vi "dfd_NStage MRate Filter Design with CIC.vi"(4 "filtering mode":T8=2 items=["No Rate Change", "Interpolation", "Decimation"], 6 "fs [Hz]":dbl=1000.0, 8 "error in (no error)":errorcluster, 9 "ripple specs":T1={"passband"=0.03624968728875148, "stopband"=0.001, "dB/linear? (T: dB)"=FALSE}, 10 "freq spec":T2={"fpass"=55.0, "fstop"=70.0}, 11 "CIC factor":i32=2) -> (0 "error out":errorcluster, 3 "multirate filters out":T3[](array[typedef]) {"mMRate_SumWl" min=1 max=32 step=1; "mMRate_InputIwl" min=1 max=32 step=1; "mMRate_GainWl" min=1 max=32 step=1; "mMRate_OutputWl" min=1 max=32 step=1; "mMRate_InputWl" min=1 max=32 step=1; "mMRate_CoefWl" min=1 max=32 step=1; "mMRate_Mode" items=["Default"=-1, "No Rate Change"=0, "Interpolation"=1, "Decimation"=2, "Interpolated"=3, "Rational"=4]})   [LabVIEW 2017, in "NI_DigFilterLicensed.lvlib"]
uses:
  <vilib>/addons/Digital Filter Design/NI_DigFilterLicensed.lvlib
  <vilib>/addons/Digital Filter Design/_Objects.llb/DFD Multirate Filtering Mode.ctl
  <vilib>/addons/Digital Filter Design/_Objects.llb/DFD Multirate Filter Obj.ctl
  <vilib>/addons/Digital Filter Design/_Objects.llb/DFD Multirate Mode.ctl
  <vilib>/addons/Digital Filter Design/_Objects.llb/DFD Coef Norm Type.ctl
  <vilib>/addons/Digital Filter Design/_Objects.llb/DFD Round-off Mode.ctl
  <vilib>/addons/Digital Filter Design/_Objects.llb/DFD FXP MRate Multiply Mode.ctl
  <vilib>/addons/Digital Filter Design/_Objects.llb/DFD Multirate Filter Specification (Design).ctl
  <vilib>/addons/Digital Filter Design/_Objects.llb/DFD Filter Ripple Specification (Design).ctl
  <vilib>/addons/Digital Filter Design/NI_DigFilter_Process.lvlib
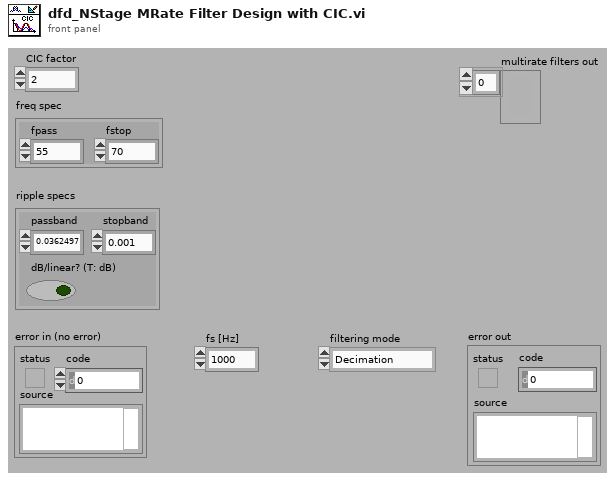
[diagram p1: front panel]
types:
  T1 = typedef "NI_DigFilterLicensed.lvlib/DFD Filter Ripple Specification (Design).ctl" = cluster{"passband":dbl, "stopband":dbl, "dB/linear? (T: dB)":bool}
  T2 = typedef "NI_DigFilterLicensed.lvlib/DFD Multirate Filter Specification (Design).ctl" = cluster{"fpass":dbl, "fstop":dbl}
  T3 = typedef "NI_DigFilterLicensed.lvlib/DFD Multirate Filter Obj.ctl" = cluster{"mMRate_Structure":enum16{"CIC", "FIR", "IIR", "Lattice"}, "mMRate_Mode":T4, "mMRate_Factor":i32, "mMRate_FIRParams":cluster{"mMRate_FIR_H":dbl[], "mMRate_FIR_IsNyquist?":bool, "mMRate_FIR_IsSymmetric?":bool}, "mMRate_CICParams":cluster{"mMRate_CIC_#Stage":i32, "mMRate_CIC_Lag":i32, "mMRate_CIC_Type":enum16{"Lowpass", "Highpass"}}, "mMRate_Order":i32, "mMRate_Version":string, "mMRate_Comments":string, "mMRate_RationalFactor":cluster{"mMRate_L":i32, "mMRate_M":i32}, "mMRate_Fs":dbl, "mMRate_Quantized?":bool, "mMRate_QFilterGain":dbl, "mMRate_CoefWl":i16, "mMRate_Scaling":cluster{"mMRate_ScaleByPowerOf2?":bool, "mMRate_ScaleType":T5}, "mMRate_InputWl":i16, "mMRate_OutputWl":i16, "mMRate_OutputMode":T6, "mMRate_MultMode":T7, "mMRate_BitPruning":bool, "mMRate_GainWl":i16, "mMRate_OutputFwl":i16, "mMRate_SumIwl":i16, "mMRate_InputIwl ":i16, "mMRate_SumWl":i16, "mMRate_CoefIwl":i16}
  T4 = typedef "NI_DigFilterLicensed.lvlib/DFD Multirate Mode.ctl" = i16
  T5 = typedef "NI_DigFilterLicensed.lvlib/DFD Coef Norm Type.ctl" = enum16{"No Norm", "Time Domain 1-Norm", "Time Domain 2-Norm", "Time Domain Inf-Norm"}
  T6 = typedef "NI_DigFilterLicensed.lvlib/DFD Round-off Mode.ctl" = enum16{"Nearest", "Truncation"}
  T7 = typedef "NI_DigFilterLicensed.lvlib/DFD FXP MRate Multiply Mode.ctl" = enum16{"Truncated", "Full"}
  T8 = typedef "NI_DigFilterLicensed.lvlib/DFD Multirate Filtering Mode.ctl" = u16
  T9 = typedef "NI_DigFilterLicensed.lvlib/DFD Filter Obj.ctl" = cluster{"mSRate_Fs":dbl, "mSRate_Version":string, "mSRate_Comments":string, "mSRate_OrgCoef":T10, "mSRate_CurCoef":T10, "mSRate_Quantized?":bool, "mSRate_QCoef":T10, "mSRate_QSettings":T12[], "mSRate_Order":i32, "mSRate_Scaling":cluster{"mSRate_ScaleByPowerOf2?":bool, "mSRate_ScaleType":T5}}
  T10 = typedef "NI_DigFilterLicensed.lvlib/DFD Filter Coef.ctl" = cluster{"type":T11, "gain":dbl, "coef a (k)":dbl[], "coef b (v)":dbl[]}
  T11 = typedef "NI_DigFilterLicensed.lvlib/DFD Filter Structure Type Selector.ctl" = enum16{"Undefined", "FIR Direct Form", "FIR Direct Form Transposed", "FIR Symmetric", "FIR Antisymmetric", "IIR Direct Form I", "IIR Direct Form I Transposed", "IIR Direct Form II", "IIR Direct Form II Transposed", "IIR Cascaded Second Order Sections Form I", "IIR Cascaded Second Order Sections Form I Transposed", "IIR Cascaded Second Order Sections Form II", "IIR Cascaded Second Order Sections Form II Transposed", "Lattice Allpass (basic sections)", "Lattice Allpass (one multiplier sections)", "Lattice Allpass (normalized sections)", "Lattice AR (basic sections)", "Lattice AR (one multiplier sections)", "Lattice AR (normalized sections)", "Lattice MA (minimum phase)", "Lattice MA (maximum phase)", "Lattice ARMA (basic sections)", "Lattice ARMA (one multiplier sections)", "Lattice ARMA (normalized sections)"}
  T12 = typedef "NI_DigFilterLicensed.lvlib/dfd_Internal Quantization Settings.ctl" = cluster{"source":T13, "wl":i16, "iwl":i16, "overflow mode":enum16{"Saturation", "Wrap"}, "rounding mode":enum16{"Nearest", "Truncation"}, "signed?":bool}
  T13 = typedef "NI_DigFilterLicensed.lvlib/dfd_Internal Quantization Srcs.ctl" = u16
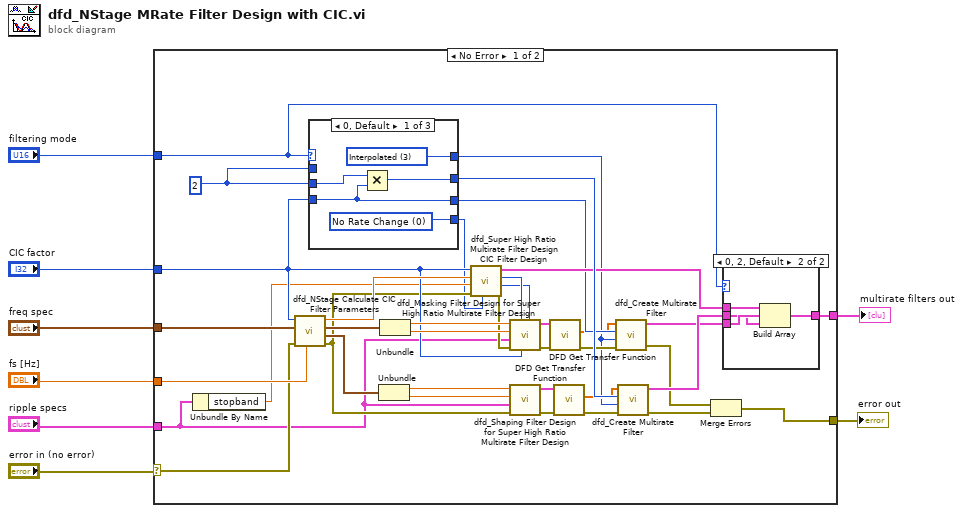
[diagram p0: block diagram]
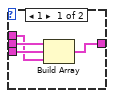
[diagram p2: hidden frame]
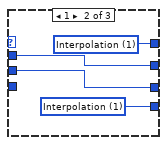
[diagram p3: hidden frame]
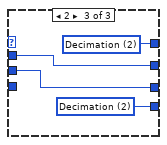
[diagram p4: hidden frame]
diagram:
  n1 = case shown="No Error" "error in (no error)" {
    selector: "error in (no error)" -> [w29 w68]
    tunnel: "fs [Hz]" -> [w46 _]
    tunnel: "ripple specs" -> [w10 _]
    tunnel: "filtering mode" -> [w32 _]
    tunnel: [w31 _] -> w7
    tunnel: "CIC factor" -> [w30 _]
    tunnel: [w17 w68] -> w4
    tunnel: "freq spec" -> [w14 _]
    frame No Error {
      w13 = 2 ("CIC factor")
      n2 = Unbundle By Name(w10) -> ("stopband"=w11:dbl)
      n3 = call <vilib>:"dfd_NStage Calculate CIC Filter Parameters.vi"("fs [Hz]"=w46, "error in (no error)"=w29, "freq spec"=w14, "CIC factor"=w30) -> ("error out"=w12:errorcluster, "shaping para"=w45:cluster{"fpass":dbl, "stop":dbl}, "masking para"=w38:cluster{"fpass":dbl, "fstop":dbl}, "CIC fstop"=w40:dbl)  [unwired: 2 in, 2 out]
      n4 = case shown="0, Default" w32 {
        tunnel: w13 -> [_ w62 w67]
        tunnel: [w57 w62 w67] -> w41
        tunnel: w13 -> [w58 w63 w66]
        tunnel: [w59 w63 w66] -> w26
        tunnel: [w55 w60 w64] -> w9
        tunnel: w30 -> [w59 _ _]
        tunnel: [w56 w61 w65] -> w21
        frame 0, Default {
          w55 = T8 0 items=["No Rate Change", "Interpolation", "Decimation"] ("filtering mode")
          w56 = T4 3 items=["Default"=-1, "No Rate Change"=0, "Interpolation"=1, "Decimation"=2, "Interpolated"=3] ("mode")
          n5 = Multiply(x=w58, y=w59) -> (x*y=w57:i32)
        }
        frame 1 {
          w60 = T8 1 items=["No Rate Change", "Interpolation", "Decimation"] ("filtering mode")
          w61 = T4 1 items=["Default"=-1, "No Rate Change"=0, "Interpolation"=1, "Decimation"=2, "Interpolated"=3] ("mode")
        }
        frame 2 {
          w64 = T8 2 items=["No Rate Change", "Interpolation", "Decimation"] ("filtering mode")
          w65 = T4 2 items=["Default"=-1, "No Rate Change"=0, "Interpolation"=1, "Decimation"=2, "Interpolated"=3] ("mode")
        }
      }
      n6 = Unbundle(w45) -> ("fpass"=w44:dbl, "stop"=w43:dbl)
      n7 = Unbundle(w38) -> ("fpass"=w37:dbl, "fstop"=w36:dbl)
      n8 = call <vilib>:"dfd_Super High Ratio Multirate Filter Design CIC Filter Design.vi"("filtering mode"=w9, "error in (no error)"=w12, "stop band attenuation [dB]"=w11, "fstop"=w40, "CIC factor"=w30) -> ("error out"=w28:errorcluster, "CIC order"=w15:i32, "CIC stage"=w39:i32, "multirate filter out"=w35:T3)  [unwired: 1 in, 2 out]
      n9 = call <vilib>:"dfd_Masking Filter Design for Super High Ratio Multirate Filter Design.vi"("CIC order"=w15, "CIC factor"=w30, "CIC stage"=w39, "error in (no error)"=w28, "ripple specs"=w10, "fstop"=w36, "fpass"=w37) -> ("error out"=w20:errorcluster, "filter out"=w24:T9)  [unwired: 1 in, 2 out]
      n10 = call <vilib>:"dfd_Shaping Filter Design for Super High Ratio Multirate Filter Design.vi"("error in (no error)"=w12, "ripple specs"=w10, "fstop"=w43, "fpass"=w44) -> ("error out"=w19:errorcluster, "filter out"=w42:T9)  [unwired: 1 in, 5 out]
      n11 = call <vilib>:"DFD Get Transfer Function.vi"("error in (no error)"=w20, "filter in"=w24) -> ("error out"=w25:errorcluster, "numerator"=w23:dbl[])  [unwired: 8 out]
      n12 = call <vilib>:"DFD Get Transfer Function.vi"("error in (no error)"=w19, "filter in"=w42) -> ("error out"=w18:errorcluster, "numerator"=w22:dbl[])  [unwired: 8 out]
      n13 = call <vilib>:"dfd_Create Multirate Filter.vi"("error in (no error)"=w25, "mode"=w21, "factor"=w26, "h (n)"=w23) -> ("error out"=w16:errorcluster, "multirate filter out"=w33:T3)  [unwired: 1 in, 5 out]
      n14 = call <vilib>:"dfd_Create Multirate Filter.vi"("error in (no error)"=w18, "mode"=w21, "factor"=w41, "h (n)"=w22) -> ("error out"=w27:errorcluster, "multirate filter out"=w34:T3)  [unwired: 1 in, 5 out]
      n15 = Merge Errors(w16, w27) -> (w17:errorcluster)
      n16 = case shown="0, 2, Default" w32 {
        tunnel: w35 -> [w48 w54]
        tunnel: w34 -> [w50 w52]
        tunnel: w33 -> [w49 w53]
        tunnel: [w47 w51] -> w31
        frame 1 {
          n17 = Build Array(w50, w49, w48) -> (w47:T3[])
        }
        frame 0, 2, Default {
          n18 = Build Array(w54, w53, w52) -> (w51:T3[])
        }
      }
    }
    frame Error {
    }
  }
  "multirate filters out" <- w7
  "error out" <- w4
